vi "Query Trigger Event Status.vi"(7 "Wait Time (10 S)":dbl=10.0, 8 "error in (no error)":errorcluster, 9 "Trigger Number (1)":i32=1, 10 "Trigger Type (5: Trigger Generator)":i32(ring)=5 items=["Digital IO", "Blender", "Timer", "TSP Link", "LAN", "Trigger Generator"], 11 "VISA resource name":refnum<visa-resource-name>) -> (0 "error out":errorcluster, 2 "Event Triggered":bool, 3 "VISA resource name out":refnum<visa-resource-name>)   [LabVIEW 2015, in "Keithley 2600 Series.lvlib"]
doc: "Indicates whether or not an event was triggered during the timeout period."
uses:
  Keithley 2600 Series.lvlib
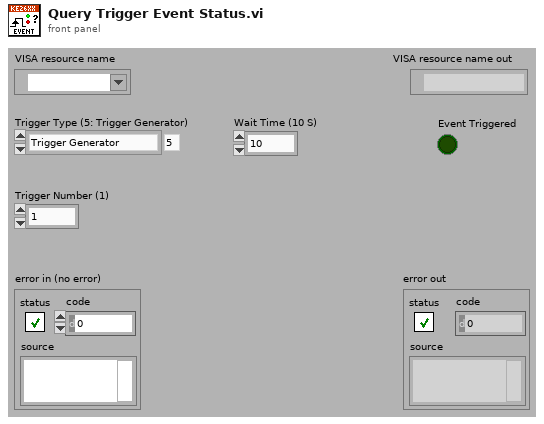
[diagram p1: front panel]
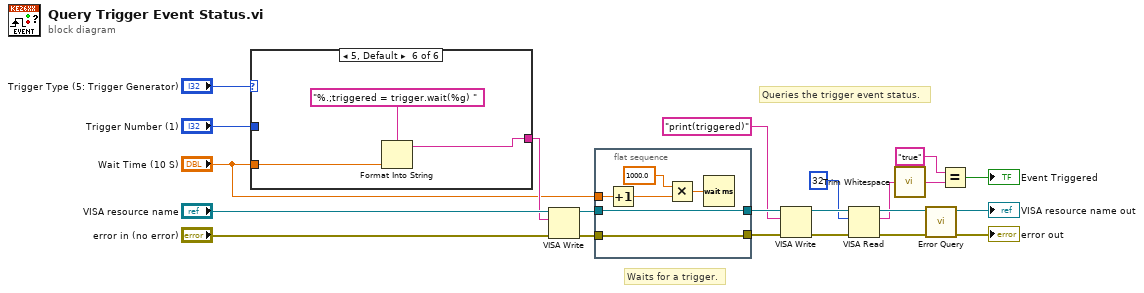
[diagram p0: block diagram]
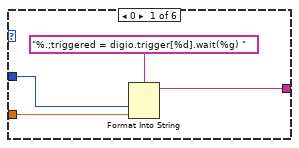
[diagram p2: hidden frame]
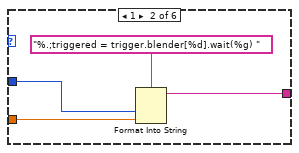
[diagram p3: hidden frame]
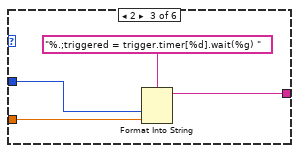
[diagram p4: hidden frame]
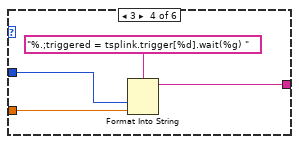
[diagram p5: hidden frame]
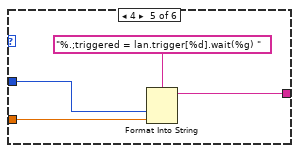
[diagram p6: hidden frame]
diagram:
  # "Queries the trigger event status."
  # "Waits for a trigger."
  n1 = case shown="5, Default" "Trigger Type (5: Trigger Generator)" {
    tunnel: "Trigger Number (1)" -> [w25 w29 w33 w37 w41 _]
    tunnel: "Wait Time (10 S)" -> [w24 w28 w32 w36 w40 w44]
    tunnel: [w23 w27 w31 w35 w39 w43] -> w2
    frame 0 {
      n2 = Format Into String(format string="%.;triggered = digio.trigger[%d].wait(%g) ", w25, w24) -> (resulting string=w23:string)  [unwired: 2 in, 1 out]
    }
    frame 1 {
      n3 = Format Into String(format string="%.;triggered = trigger.blender[%d].wait(%g) ", w29, w28) -> (resulting string=w27:string)  [unwired: 2 in, 1 out]
    }
    frame 2 {
      n4 = Format Into String(format string="%.;triggered = trigger.timer[%d].wait(%g) ", w33, w32) -> (resulting string=w31:string)  [unwired: 2 in, 1 out]
    }
    frame 3 {
      n5 = Format Into String(format string="%.;triggered = tsplink.trigger[%d].wait(%g) ", w37, w36) -> (resulting string=w35:string)  [unwired: 2 in, 1 out]
    }
    frame 4 {
      n6 = Format Into String(format string="%.;triggered = lan.trigger[%d].wait(%g) ", w41, w40) -> (resulting string=w39:string)  [unwired: 2 in, 1 out]
    }
    frame 5, Default {
      n7 = Format Into String(format string="%.;triggered = trigger.wait(%g) ", w44) -> (resulting string=w43:string)  [unwired: 2 in, 1 out]
    }
  }
  n8 = VISA Write(VISA resource name="VISA resource name", write buffer=w2, error in (no error)="error in (no error)") -> (VISA resource name out=w4:refnum<visa-resource-name>, error out=w3:errorcluster)  [unwired: 1 out]
  n9 = flat-sequence {
    tunnel: w4 -> [w51]
    tunnel: w3 -> [w50]
    tunnel: [w51] -> w9
    tunnel: [w50] -> w8
    tunnel: "Wait Time (10 S)" -> [w47]
    frame #0 {
      n10 = Increment(x=w47) -> (x+1=w46:dbl)
      n11 = Multiply(x=1000.0, y=w46) -> (x*y=w49:dbl)
      n12 = Wait (ms)(milliseconds to wait=w49) -> ()  [unwired: 1 out]
    }
  }
  n13 = VISA Write(VISA resource name=w9, write buffer="print(triggered)" ("format string"), error in (no error)=w8) -> (VISA resource name out=w18:refnum<visa-resource-name>, error out=w16:errorcluster)  [unwired: 1 out]
  n14 = VISA Read(VISA resource name=w18, byte count=u32 32, error in (no error)=w16) -> (VISA resource name out=w17:refnum<visa-resource-name>, read buffer=w13:string, error out=w15:errorcluster)  [unwired: 1 out]
  n15 = call <vilib>:"Trim Whitespace.vi"("string"=w13) -> ("trimmed string"=w11:string)  [unwired: 1 in]
  n16 = call "Error Query.vi"("error in (no error)"=w15, "VISA resource name"=w17) -> ("error out"=→"error out":errorcluster, "VISA resource name out"=→"VISA resource name out":refnum<visa-resource-name>)  [unwired: 6 in, 2 out]
  n17 = Equal?(x="true", y=w11) -> (x = y?=→"Event Triggered":bool)
